vi "H5Pget_fapl_core.vi"(6 "error in (no error)":errorcluster, 9 "HDF5 Property List Ref":T1) -> (0 "error out":errorcluster, 1 "Backing Store":bool, 2 "Increment":u32, 3 "HDF5 Property List Ref out":T1)   [LabVIEW 2017]
doc: "Queries core file driver properties."
uses:
  <vilib>/UPVI/lvhdf5/library.llb/HDF5 Ref.ctl
  <vilib>/UPVI/lvhdf5/hdf5.dll
panel:
  # "LVHDF5 Toolkit\nCopyright (c) 2005-2013 by Jason D. Sommerville\nCopyright (c) 2014 by UPVI, LLC.\n\nThis use and distribution of this file is governed by the terms found in \nLICENSE.txt distributed with this toolkit and installed at\n <user.lib>\\_lvhdf5\\LICENSE.txt"
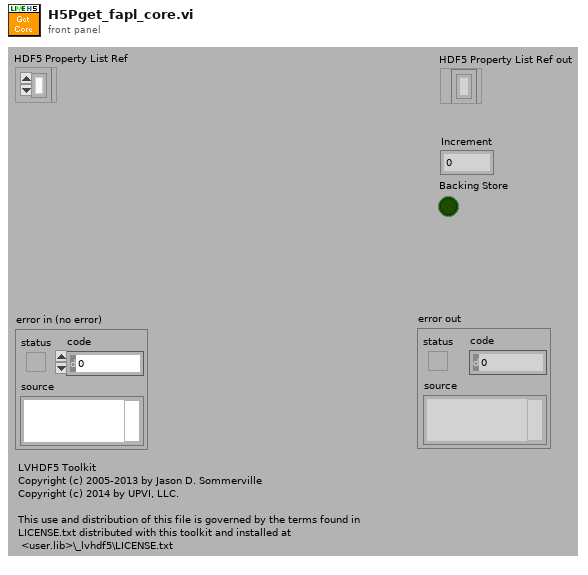
[diagram p1: front panel]
types:
  T1 = typedef "HDF5 Ref.ctl" = refnum<k1>
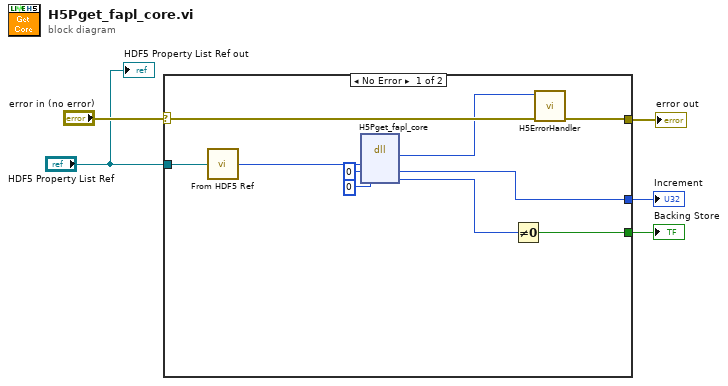
[diagram p0: block diagram]
diagram:
  n1 = case shown="No Error" "error in (no error)" {
    selector: "error in (no error)" -> [w15 w16]
    tunnel: [w14 w16] -> w4
    tunnel: "HDF5 Property List Ref" -> [w13 _]
    tunnel: [w8 _] -> w2
    tunnel: [w6 _] -> w1
    frame No Error {
      n2 = call <vilib>:"From HDF5 Ref.vi"("HDF5 Ref"=w13) -> ("I32"=w12:i32)
      n3 = dll-call lib="C:/Program Files/National Instruments/LabVIEW 2017/vi.lib/UPVI/lvhdf5/hdf5.dll" fn="H5Pget_fapl_core"("plist_id"=w12, "increment"=u32 0, "backing_store"=0) -> ("return type"=w11:i32, "increment"=w8:u64, "backing_store"=w7:i32)  [unwired: 4 in, 2 out]
      n4 = Not Equal To 0?(x=w7) -> (x != 0?=w6:bool)
      n5 = call <vilib>:"H5ErrorHandler.vi"("error in (no error)"=w15, "herr_t"=w11) -> ("error out"=w14:errorcluster)  [unwired: 3 in, 4 out]
    }
    frame Error {
    }
  }
  "error out" <- w4
  "Increment" <- w2
  "Backing Store" <- w1
  "HDF5 Property List Ref out" <- "HDF5 Property List Ref"
